vi "Round 3.vi"(8 "error in (no error)":errorcluster, 11 "KNR in":T1) -> (0 "error out":errorcluster, 3 "KNR out":T1)   [LabVIEW 2013]
uses:
  <userlib>/KNR OS 3.0 LabVIEW Toolkit/Type Definition/KNR3 Reference.ctl
  <userlib>/_FPGA Interface Advanced Tools/FPGA Interface Base/FPGA Interface Base.lvclass
  <userlib>/KNR OS 3.0 LabVIEW Toolkit/Type Definition/Resource.ctl
  <userlib>/KNR OS 3.0 LabVIEW Toolkit/Type Definition/DC Motor Port.ctl
  Global 1.vi
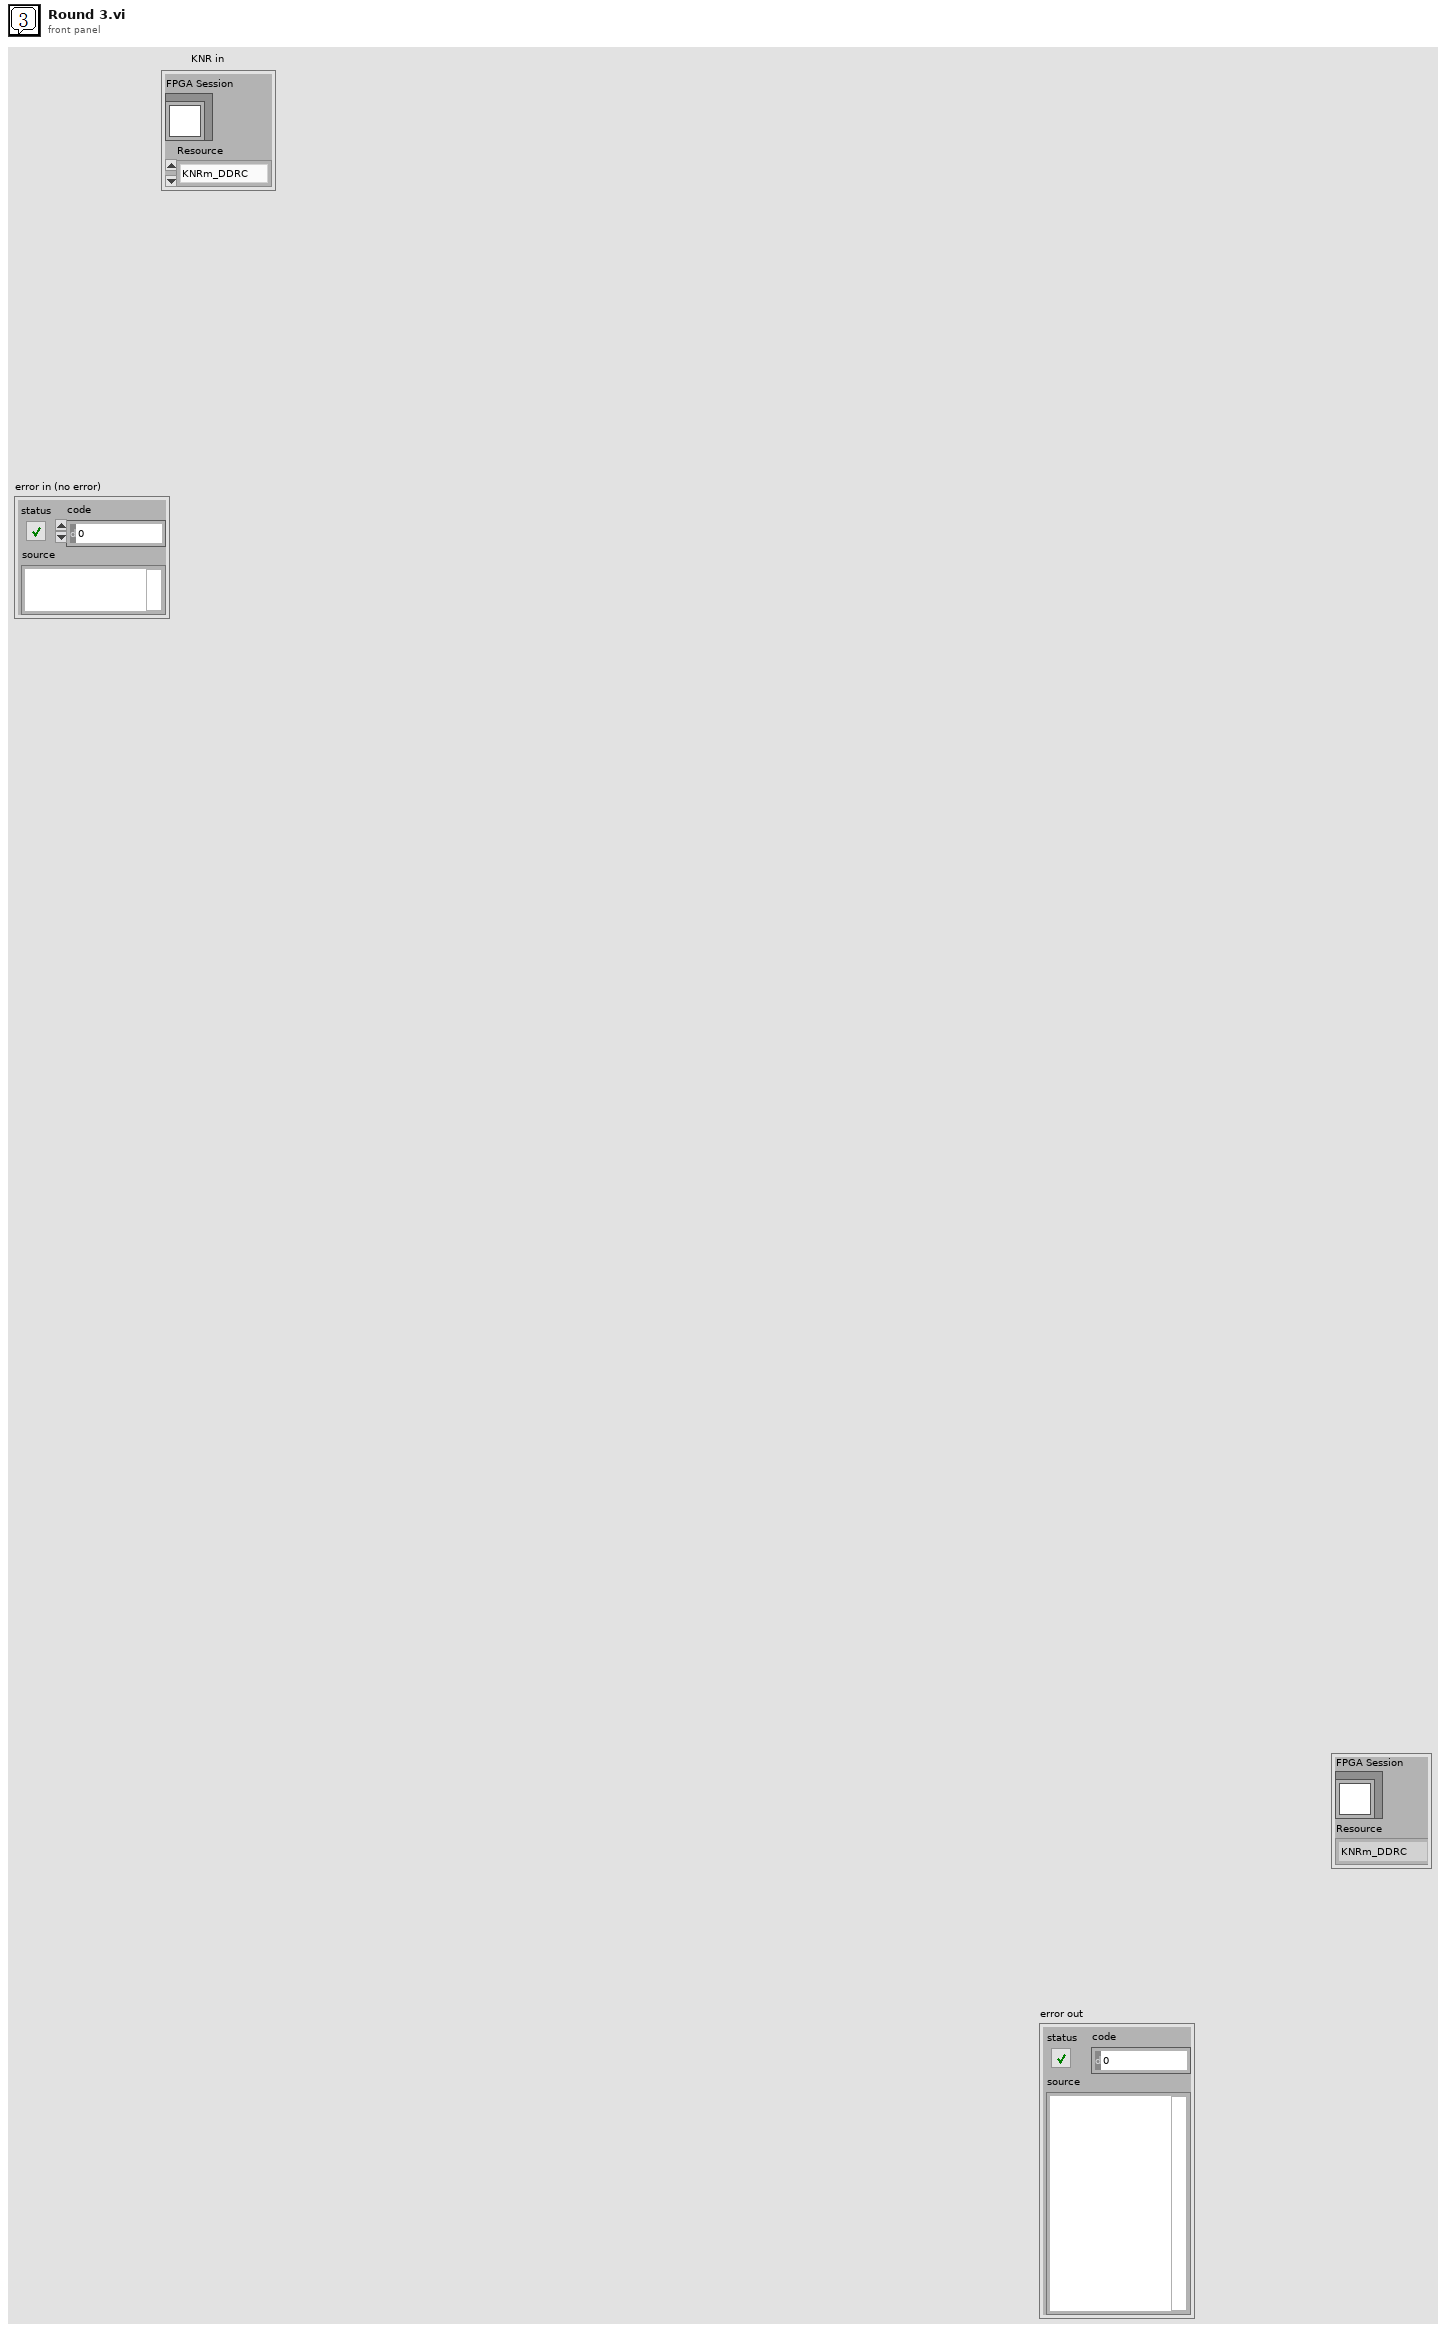
[diagram p1: front panel]
types:
  T1 = typedef "KNR3 Reference.ctl" = cluster{"FPGA Session":refnum<class "FPGA Interface Base.lvclass">, "Resource":T2}
  T2 = typedef "Resource.ctl" = enum16{"KNRm_DDRC", "KNRm_DDDD", "KNRm_DDDR", "KNRm_DDDC", "KNR"}
  T3 = typedef "DC Motor Port.ctl" = u16
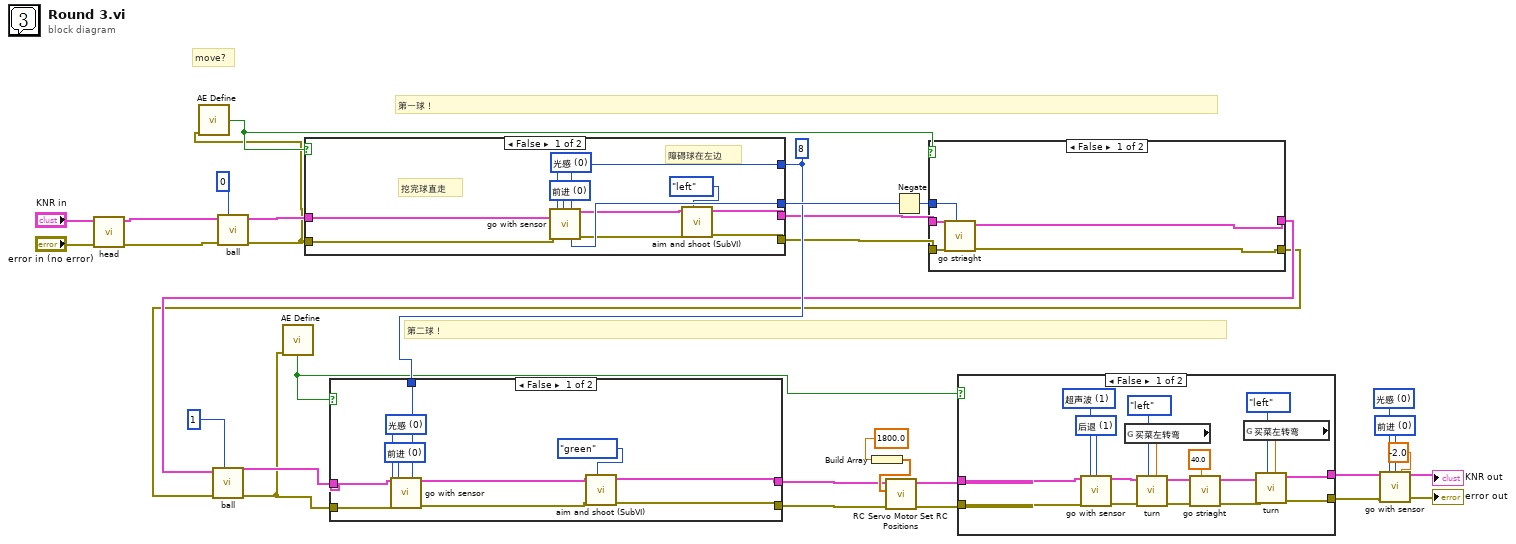
[diagram p0: block diagram]
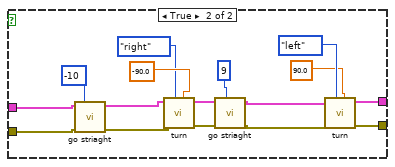
[diagram p2: hidden frame]
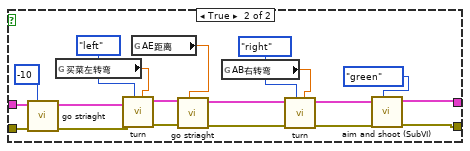
[diagram p3: hidden frame]
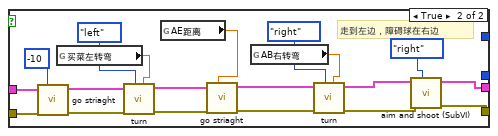
[diagram p4: hidden frame]
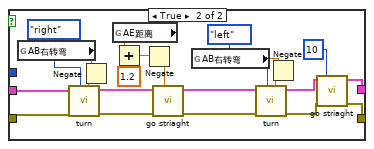
[diagram p5: hidden frame]
diagram:
  w21 = 8
  w27 = T3 0 items=["前进", "后退"] ("方向")
  w28 = T3 0 items=["光感", "超声波"] ("传感器类型")
  # "move?"
  # "第二球！"
  # "第一球！"
  n1 = call "head.vi"("error in (no error)"="error in (no error)", "KNR in"="KNR in") -> ("error out"=w1:errorcluster, "KNR out"=w2:T1)  [unwired: 8 in]
  n2 = call "ball.vi"("Numeric"=0, "error in (no error)"=w1, "KNR in"=w2) -> ("error out"=w19:errorcluster, "KNR out"=w25:T1)  [unwired: 6 in, 1 out]
  n3 = call "AE Define.vi"("error in"=w19) -> ("move?"=w20:bool)  [unwired: 2 in, 1 out]
  n4 = case shown="False" w20 {
    tunnel: w25 -> [w41 w51]
    tunnel: w19 -> [w40 w50]
    tunnel: [w35 w45] -> w10
    tunnel: [w33 w44] -> w9
    tunnel: w21 -> [w39 _]
    tunnel: [w38 _] -> w22
    frame False {
      w42 = T3 0 items=["前进", "后退"] ("方向")
      w43 = T3 0 items=["光感", "超声波"] ("传感器类型")
      # "障碍球在左边"
      # "挖完球直走"
      n5 = call "go with sensor.vi"("KNR in"=w41, "传感器类型"=w43, "方向"=w42, "then go:"=w39, "error in (no error)"=w40) -> ("KNR out"=w36:T1, "offset"=w38:i32, "error out"=w34:errorcluster)  [unwired: 8 in]
      n6 = call "aim and shoot (SubVI).vi"("pin"=enum16{"white", "green", "left", "right"}."left", "error in (no error)"=w34, "KNR in"=w36) -> ("error out"=w33:errorcluster, "KNR out"=w35:T1)  [unwired: 7 in]
    }
    frame True {
      # "走到左边，障碍球在右边"
      n7 = call "go striaght.vi"("距离"=-10, "error in (no error)"=w50, "KNR in"=w51) -> ("error out"=w52:errorcluster, "KNR out"=w53:T1)  [unwired: 7 in]
      n8 = global read "Global 1.vi" "买菜左转弯"() -> (w61:dbl)
      n9 = call "turn.vi"("Angle"=w61, "side"=enum16{"right", "left"}."left", "error in (no error)"=w52, "KNR in"=w53) -> ("error out"=w54:errorcluster, "KNR out"=w55:T1)  [unwired: 6 in]
      n10 = global read "Global 1.vi" "AE距离"() -> (w58:dbl)
      n11 = call "go striaght.vi"("距离"=w58, "error in (no error)"=w54, "KNR in"=w55) -> ("error out"=w56:errorcluster, "KNR out"=w57:T1)  [unwired: 7 in]
      n12 = global read "Global 1.vi" "AB右转弯"() -> (w60:dbl)
      n13 = call "turn.vi"("Angle"=w60, "side"=enum16{"right", "left"}."right", "error in (no error)"=w56, "KNR in"=w57) -> ("error out"=w46:errorcluster, "KNR out"=w47:T1)  [unwired: 6 in]
      n14 = call "aim and shoot (SubVI).vi"("pin"=enum16{"white", "green", "left", "right"}."right", "error in (no error)"=w46, "KNR in"=w47) -> ("error out"=w44:errorcluster, "KNR out"=w45:T1)  [unwired: 7 in]
    }
  }
  n15 = Build Array(1800.0 ("element")) -> (w31:dbl[])
  n16 = Negate(x=w22) -> (-x=w23:i32)
  n17 = case shown="False" w20 {
    tunnel: [w64 w71] -> w17
    tunnel: [w63 w70] -> w16
    tunnel: w10 -> [w67 w80]
    tunnel: w9 -> [w66 w79]
    tunnel: w23 -> [w65 _]
    frame False {
      n18 = call "go striaght.vi"("距离"=w65, "error in (no error)"=w66, "KNR in"=w67) -> ("error out"=w63:errorcluster, "KNR out"=w64:T1)  [unwired: 7 in]
    }
    frame True {
      n19 = global read "Global 1.vi" "AB右转弯"() -> (w88:dbl)
      n20 = Negate(x=w88) -> (-x=w86:dbl)
      n21 = call "turn.vi"("Angle"=w86, "side"=enum16{"right", "left"}."right", "error in (no error)"=w79, "KNR in"=w80) -> ("error out"=w84:errorcluster, "KNR out"=w85:T1)  [unwired: 6 in]
      n22 = global read "Global 1.vi" "AE距离"() -> (w74:dbl)
      n23 = Add(x=w74, y=1.2) -> (x+y=w73:dbl)
      n24 = Negate(x=w73) -> (-x=w76:dbl)
      n25 = call "go striaght.vi"("距离"=w76, "error in (no error)"=w84, "KNR in"=w85) -> ("error out"=w81:errorcluster, "KNR out"=w82:T1)  [unwired: 7 in]
      n26 = global read "Global 1.vi" "AB右转弯"() -> (w78:dbl)
      n27 = Negate(x=w78) -> (-x=w77:dbl)
      n28 = call "turn.vi"("Angle"=w77, "side"=enum16{"right", "left"}."left", "error in (no error)"=w81, "KNR in"=w82) -> ("error out"=w68:errorcluster, "KNR out"=w69:T1)  [unwired: 6 in]
      n29 = call "go striaght.vi"("距离"=10, "error in (no error)"=w68, "KNR in"=w69) -> ("error out"=w70:errorcluster, "KNR out"=w71:T1)  [unwired: 7 in]
    }
  }
  n30 = call "ball.vi"("Numeric"=1, "error in (no error)"=w16, "KNR in"=w17) -> ("error out"=w3:errorcluster, "KNR out"=w18:T1)  [unwired: 6 in, 1 out]
  n31 = call "AE Define.vi"("error in"=w3) -> ("move?"=w6:bool)  [unwired: 2 in, 1 out]
  n32 = case shown="False" w6 {
    tunnel: w3 -> [w96 w105]
    tunnel: [w91 w102] -> w8
    tunnel: [w90 w100] -> w7
    tunnel: w21 -> [w95 _]
    tunnel: w18 -> [w89 w99]
    frame False {
      w98 = T3 0 items=["前进", "后退"] ("方向")
      w97 = T3 0 items=["光感", "超声波"] ("传感器类型")
      n33 = call "go with sensor.vi"("KNR in"=w89, "传感器类型"=w97, "方向"=w98, "then go:"=w95, "error in (no error)"=w96) -> ("KNR out"=w93:T1, "error out"=w92:errorcluster)  [unwired: 8 in, 1 out]
      n34 = call "aim and shoot (SubVI).vi"("pin"=enum16{"white", "green", "left", "right"}."green", "error in (no error)"=w92, "KNR in"=w93) -> ("error out"=w90:errorcluster, "KNR out"=w91:T1)  [unwired: 7 in]
    }
    frame True {
      n35 = call "go striaght.vi"("距离"=-10, "error in (no error)"=w105, "KNR in"=w99) -> ("error out"=w106:errorcluster, "KNR out"=w107:T1)  [unwired: 7 in]
      n36 = global read "Global 1.vi" "买菜左转弯"() -> (w116:dbl)
      n37 = call "turn.vi"("Angle"=w116, "side"=enum16{"right", "left"}."left", "error in (no error)"=w106, "KNR in"=w107) -> ("error out"=w109:errorcluster, "KNR out"=w110:T1)  [unwired: 6 in]
      n38 = global read "Global 1.vi" "AE距离"() -> (w113:dbl)
      n39 = call "go striaght.vi"("距离"=w113, "error in (no error)"=w109, "KNR in"=w110) -> ("error out"=w111:errorcluster, "KNR out"=w112:T1)  [unwired: 7 in]
      n40 = global read "Global 1.vi" "AB右转弯"() -> (w115:dbl)
      n41 = call "turn.vi"("Angle"=w115, "side"=enum16{"right", "left"}."right", "error in (no error)"=w111, "KNR in"=w112) -> ("error out"=w101:errorcluster, "KNR out"=w103:T1)  [unwired: 6 in]
      n42 = call "aim and shoot (SubVI).vi"("pin"=enum16{"white", "green", "left", "right"}."green", "error in (no error)"=w101, "KNR in"=w103) -> ("error out"=w100:errorcluster, "KNR out"=w102:T1)  [unwired: 7 in]
    }
  }
  n43 = call <userlib>:"RC Servo Motor Set RC Positions.vi"("error in (no error)"=w7, "RC Pulse Width (1500 uS)"=w31, "KNR in"=w8) -> ("error out"=w29:errorcluster, "KNR out"=w30:T1)  [unwired: 7 in]
  n44 = case shown="False" w6 {
    tunnel: w30 -> [w132 w138]
    tunnel: w29 -> [w131 w135]
    tunnel: [w119 w144] -> w5
    tunnel: [w118 w143] -> w4
    frame False {
      w133 = T3 1 items=["前进", "后退"] ("方向")
      w134 = T3 1 items=["光感", "超声波"] ("传感器类型")
      n45 = call "go with sensor.vi"("KNR in"=w132, "传感器类型"=w134, "方向"=w133, "error in (no error)"=w131) -> ("KNR out"=w128:T1, "error out"=w127:errorcluster)  [unwired: 9 in, 1 out]
      n46 = global read "Global 1.vi" "买菜左转弯"() -> (w129:dbl)
      n47 = call "turn.vi"("Angle"=w129, "side"=enum16{"right", "left"}."left", "error in (no error)"=w127, "KNR in"=w128) -> ("error out"=w126:errorcluster, "KNR out"=w125:T1)  [unwired: 6 in]
      n48 = call "go striaght.vi"("距离"=40.0, "error in (no error)"=w126, "KNR in"=w125) -> ("error out"=w120:errorcluster, "KNR out"=w121:T1)  [unwired: 7 in]
      n49 = global read "Global 1.vi" "买菜左转弯"() -> (w122:dbl)
      n50 = call "turn.vi"("Angle"=w122, "side"=enum16{"right", "left"}."left", "error in (no error)"=w120, "KNR in"=w121) -> ("error out"=w118:errorcluster, "KNR out"=w119:T1)  [unwired: 6 in]
    }
    frame True {
      n51 = call "go striaght.vi"("距离"=-10, "error in (no error)"=w135, "KNR in"=w138) -> ("error out"=w136:errorcluster, "KNR out"=w137:T1)  [unwired: 7 in]
      n52 = call "turn.vi"("Angle"=-90.0, "side"=enum16{"right", "left"}."right", "error in (no error)"=w136, "KNR in"=w137) -> ("error out"=w146:errorcluster, "KNR out"=w147:T1)  [unwired: 6 in]
      n53 = call "go striaght.vi"("距离"=9, "error in (no error)"=w146, "KNR in"=w147) -> ("error out"=w141:errorcluster, "KNR out"=w142:T1)  [unwired: 7 in]
      n54 = call "turn.vi"("Angle"=90.0, "side"=enum16{"right", "left"}."left", "error in (no error)"=w141, "KNR in"=w142) -> ("error out"=w143:errorcluster, "KNR out"=w144:T1)  [unwired: 6 in]
    }
  }
  n55 = call "go with sensor.vi"("KNR in"=w5, "传感器类型"=w28, "方向"=w27, "then go:"=-2.0, "error in (no error)"=w4) -> ("KNR out"=→"KNR out":T1, "error out"=→"error out":errorcluster)  [unwired: 8 in, 1 out]
